vi "test Close References.vi"(8 "error in":errorcluster) -> (0 "error out":errorcluster)   [LabVIEW 2020, in "serenial.io-ase.test.lvlib"]
uses:
  serenial.io-ase.test.lvlib
  serenial.io-ase/ase/Event References.ctl
  serenial.io-ase/ase/Standard Output.ctl
  serenial.io-ase/ase/Standard Error.ctl
  serenial.io-ase/ase/Did Exit.ctl
  <vilib>/addons/_JKI Toolkits/Caraya/classes/Assert/Assert Not Error.vi
  <vilib>/addons/_JKI Toolkits/Caraya/classes/Test/Test.lvclass
  <vilib>/addons/_JKI Toolkits/Caraya/classes/Assert/Assert.lvclass
  serenial.io-ase/ase/ase.lvclass
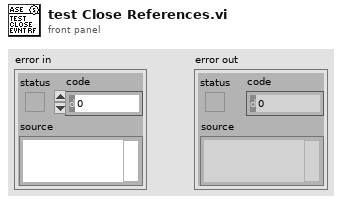
[diagram p1: front panel]
types:
  T1 = typedef "serenial.io-ase.lvlib/ase.lvclass/Event References.ctl" = cluster{"Standard Output":refnum<user-event>, "Standard Error":refnum<user-event>, "Did Exit":refnum<user-event>}
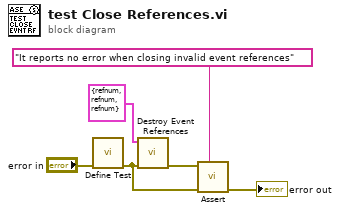
[diagram p0: block diagram]
diagram:
  n1 = call <vilib>:"Define Test.vi"("error in (no error)"="error in") -> ("error out"=w1:errorcluster)  [unwired: 10 in]
  n2 = call "Destroy Event References.vi"("error in"=w1, "Event References"=T1 {"Standard Output"=refnum, "Standard Error"=refnum, "Did Exit"=refnum}) -> ("error out"=w2:errorcluster)  [unwired: 9 in]
  n3 = call-poly <vilib>:"Assert.vi"("Label"="It reports no error when closing invalid event references", "error in (no error)"=w1, "Not Error?"=w2) -> ("error out"=→"error out":errorcluster)  [unwired: 8 in]
